vi "Control - Set User Object Tag.vi"(8 "error in (no error)":errorcluster, 11 "Folder Path":path) -> (0 "error out":errorcluster)   [LabVIEW 2017]
uses:
  <vilib>/UserTags/UserTags.lvlib
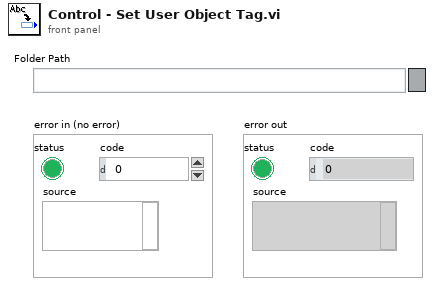
[diagram p1: front panel]
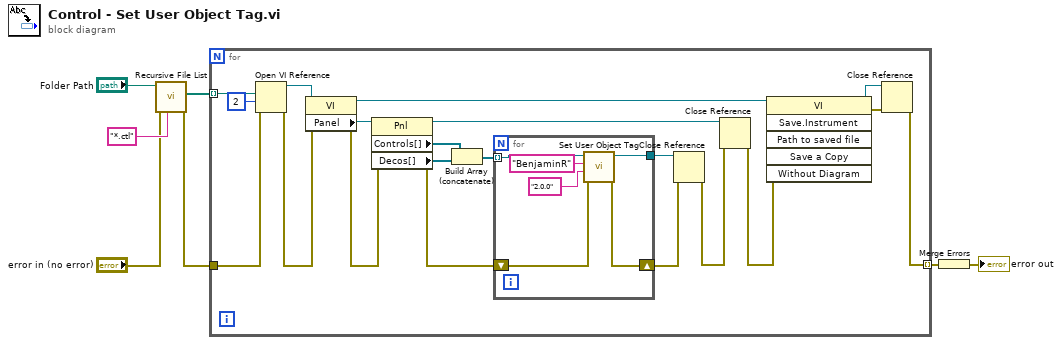
[diagram p0: block diagram]
diagram:
  n1 = call <vilib>:"Recursive File List.vi"("pattern"="*.ctl", "error in (no error)"="error in (no error)", "Folder Path"="Folder Path") -> ("error out"=w3:errorcluster, "All Files in Dir"=w4:path[])  [unwired: 4 in, 3 out]
  n2 = for {
    tunnel: w4 -> [w27] mode=indexing
    tunnel: w3 -> [w21]
    tunnel: [w16] -> w2 mode=indexing
    n3 = Open VI Reference(vi path=w27, options=2, error in (no error)=w21) -> (vi reference=w25:refnum<vi>, error out=w24:errorcluster)  [unwired: 3 in]
    n4 = property class="VI"(reference=w25, error in=w24) -> (reference out=w11:refnum<vi>, error out=w22:errorcluster, "Panel"=w23:refnum<vi>)
    n5 = property class="Pnl"(reference=w23, error in=w22) -> (reference out=w20:refnum<vi>, error out=w14:errorcluster, "Controls[]"=w8:refnum<vi>[], "Decos[]"=w10:refnum<vi>[])
    n6 = Build Array (concatenate)(w8, w10) -> (w9:refnum<vi>[])
    n7 = for {
      tunnel: [w29] -> w13
      shift-right: [w33] -> w15
      shift-left: w14 -> [w32]
      tunnel: w9 -> [w28] mode=indexing
      n8 = call <vilib>:"Set User Object Tag.vi"("error in (no error)"=w32, "Value"="2.0.0" ("Tag Name"), "Tag Name"="BenjaminR", "Generic Refnum"=w28) -> ("error out"=w33:errorcluster, "dup Generic Refnum"=w29:refnum<vi>)  [unwired: 5 in, 1 out]
    }
    n9 = Close Reference(reference=w13, error in (no error)=w15) -> (error out=w19:errorcluster)
    n10 = Close Reference(reference=w20, error in (no error)=w19) -> (error out=w12:errorcluster)
    n11 = invoke class="VI" method="Save.Instrument"(reference=w11, error in=w12) -> (reference out=w18:refnum<vi>, error out=w17:errorcluster)  [unwired: 4 in, 4 out]
    n12 = Close Reference(reference=w18, error in (no error)=w17) -> (error out=w16:errorcluster)
  }
  n13 = Merge Errors(w2) -> (→"error out":errorcluster)
